vi "BuildPieceMap.vi"(8 "error in (no error)":errorcluster, 10 "pieceArray":refnum<class "Piece.lvclass">[][](array[class]), 11 "object in":refnum<class "Board.lvclass">) -> (0 "error out":errorcluster, 3 "object out":refnum<class "Board.lvclass">)   [LabVIEW 2020, in "Board.lvclass"]
uses:
  Board.lvclass
  Pieces/Piece.lvclass
  Pieces/typedefs/pieceMap.ctl
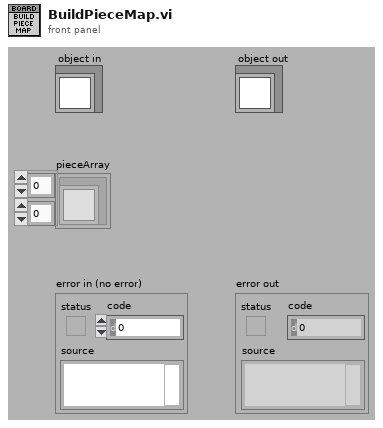
[diagram p1: front panel]
types:
  T1 = typedef "Board.lvclass/pieceMap.ctl" = map{map{string, i32}, refnum<class "Piece.lvclass">}
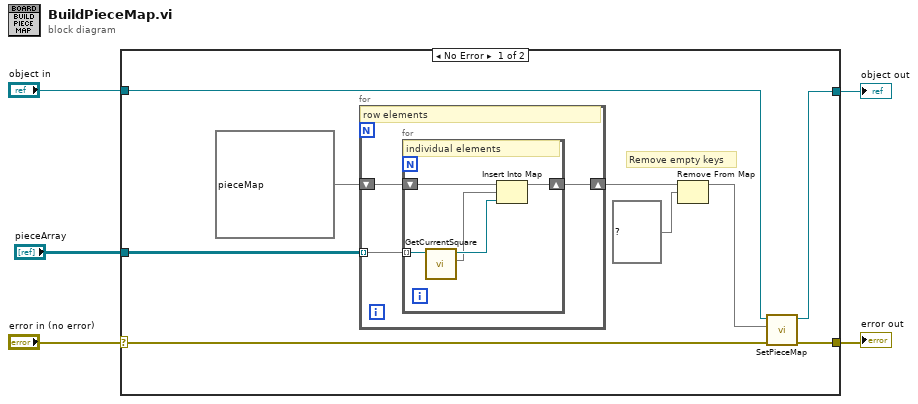
[diagram p0: block diagram]
diagram:
  n1 = case shown="No Error" "error in (no error)" {
    selector: "error in (no error)" -> [w12 w24]
    tunnel: [w11 w24] -> w4
    tunnel: [w13 w23] -> w2
    tunnel: "object in" -> [w14 w23]
    tunnel: "pieceArray" -> [w6 _]
    frame No Error {
      # "Remove empty keys"
      n2 = for {
        shift-right: [w16] -> w10
        shift-left: T1 {} ("pieceMap") -> [w17]
        tunnel: w6 -> [w15] mode=indexing
        # "row elements"
        n3 = for {
          shift-right: [w19] -> w16
          shift-left: w17 -> [w22]
          tunnel: w15 -> [w21] mode=indexing
          # "individual elements"
          n4 = call "GetCurrentSquare.vi"("object in"=w21) -> ("currentSquare"=w18:map{string, i32}, "object out"=w20:refnum<class "Piece.lvclass">)  [unwired: 5 in, 4 out]
          n5 = Insert Into Map(map in=w22, key=w18, value=w20) -> (map out=w19:T1)  [unwired: 2 out]
        }
      }
      n6 = Remove From Map(10:map{string, i32} {} ("key"), 11:w10) -> (3:w7:T1)  [unwired: 2 out]
      n7 = call "SetPieceMap.vi"("error in (no error)"=w12, "pieceMap"=w7, "object in"=w14) -> ("error out"=w11:errorcluster, "object out"=w13:refnum<class "Board.lvclass">)  [unwired: 7 in]
    }
    frame Error {
    }
  }
  "error out" <- w4
  "object out" <- w2
